vi "BallRollTime.vi"(6 "v_ini":dbl, 8 "error in (no error)":errorcluster, 9 "distance":dbl, 10 "Ball":refnum<class "Ball.lvclass">, 11 "Utilities in":refnum<class "Utilities.lvclass">) -> (0 "error out":errorcluster, 2 "time":dbl, 3 "Utilities out":refnum<class "Utilities.lvclass">)   [LabVIEW 2023, in "Utilities.lvclass"]
uses:
  Utilities.lvclass
  Ball_class/Ball.lvclass
  Ball_class/Ball.lvclass/Ball.ctl
  Ball_class/Read acc_roll.vi
  Ball_class/Read acc_slide.vi
  Ball_class/Read k_switch.vi
  Ball_class/Read velocityNorm.vi
  <vilib>/Analysis/_algsub.llb/Vector Norm.vi
  <vilib>/Analysis/_algsub.llb/Real Vector Norm.vi
panel:
  in  "k_switch":dbl=0.7142857142857143
  in  "acc_slide":dbl=-2.5
  in  "acc_roll":dbl=-0.3
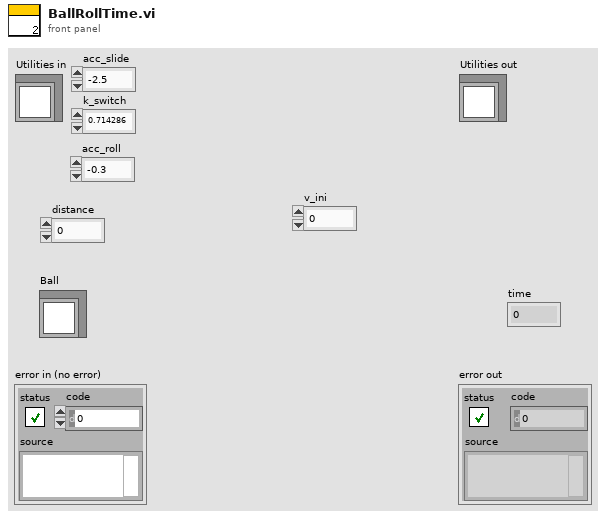
[diagram p1: front panel]
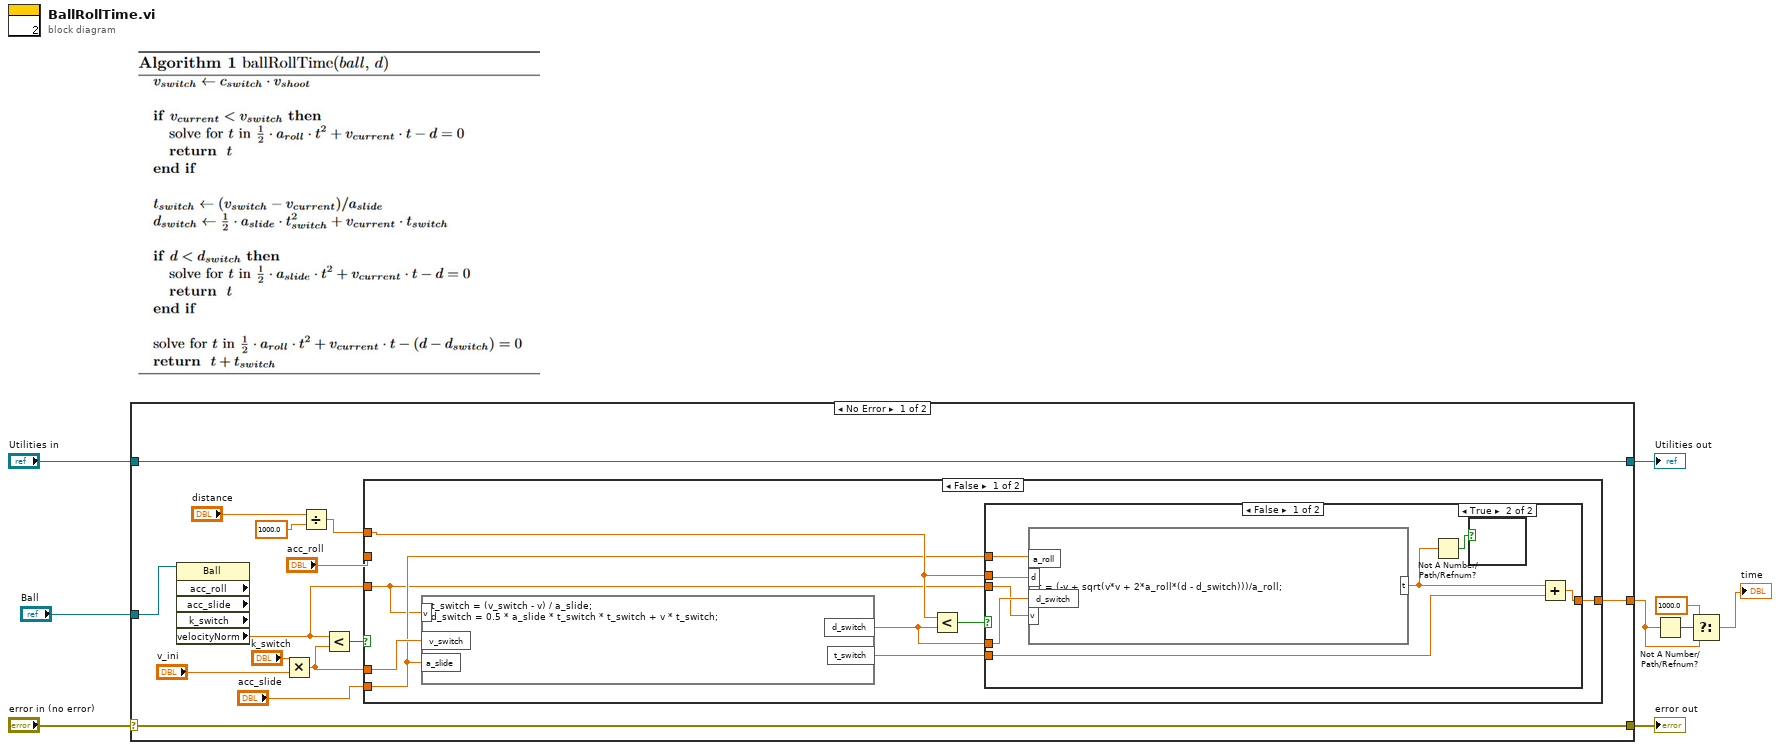
[diagram p0: block diagram]
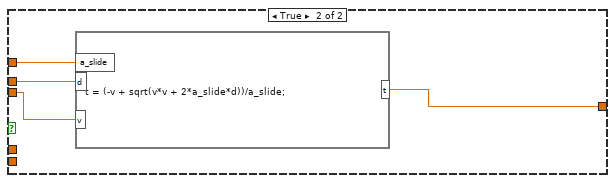
[diagram p3: hidden frame]
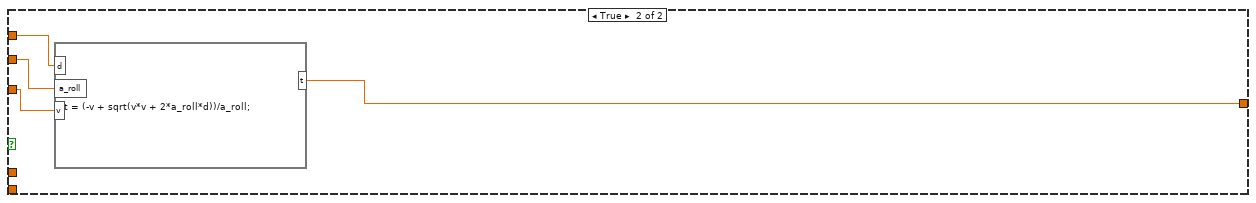
[diagram p4: hidden frame]
diagram:
  n1 = case shown="No Error" "error in (no error)" {
    selector: "error in (no error)" -> [w22 w49]
    tunnel: [w22 w49] -> w8
    tunnel: [w23 w48] -> w6
    tunnel: "Utilities in" -> [w23 w48]
    tunnel: "Ball" -> [w21 _]
    tunnel: [w19 _] -> w2
    frame No Error {
      n2 = property class="Ball" props=["acc_roll", "acc_slide", "k_switch", "velocityNorm"](reference=w21) -> ("velocityNorm"=w18:dbl)  [unwired: 1 in, 5 out]
      n3 = Multiply(x="k_switch", y="v_ini") -> (x*y=w17:dbl)
      n4 = Divide(x="distance", y=1000.0) -> (x/y=w16:dbl)
      n5 = Less?(x=w18, y=w17) -> (x < y?=w20:bool)
      n6 = case shown="False" w20 {
        tunnel: w18 -> [w24 w47]
        tunnel: "acc_roll" -> [_ w46]
        tunnel: w16 -> [w29 w45]
        tunnel: [w28 w44] -> w19
        tunnel: w17 -> [w31 _]
        tunnel: "acc_slide" -> [w27 _]
        frame False {
          n7 = formula code="t_switch = (v_switch - v) / a_slide;\nd_switch = 0.5 * a_slide * t_switch * t_switch + v * t_switch;"("v_switch"=w31, "a_slide"=w27, "v"=w24) -> ("t_switch"=w25:dbl, "d_switch"=w26:dbl)
          n8 = Less?(x=w29, y=w26) -> (x < y?=w30:bool)
          n9 = case shown="False" w30 {
            tunnel: w29 -> [w38 w43]
            tunnel: w27 -> [w37 w42]
            tunnel: w24 -> [w36 w41]
            tunnel: [w34 w40] -> w28
            tunnel: w26 -> [w39 _]
            tunnel: w25 -> [w35 _]
            frame False {
              n10 = formula code="t = (-v + sqrt(v*v + 2*a_roll*(d - d_switch)))/a_roll;"("v"=w36, "a_roll"=w37, "d"=w38, "d_switch"=w39) -> ("t"=w33:dbl)
              n11 = Not A Number/Path/Refnum?(number/path/refnum=w33) -> (NaN/Path/Refnum?=w32:bool)
              n12 = case shown="True" w32 {
                frame False {
                }
                frame True {
                }
              }
              n13 = Add(x=w33, y=w35) -> (x+y=w34:dbl)
            }
            frame True {
              n14 = formula code="t = (-v + sqrt(v*v + 2*a_slide*d))/a_slide;"("v"=w41, "a_slide"=w42, "d"=w43) -> ("t"=w40:dbl)
            }
          }
        }
        frame True {
          n15 = formula code="t = (-v + sqrt(v*v + 2*a_roll*d))/a_roll;"("v"=w47, "a_roll"=w46, "d"=w45) -> ("t"=w44:dbl)
        }
      }
    }
    frame Error {
    }
  }
  "error out" <- w8
  "Utilities out" <- w6
  n16 = Not A Number/Path/Refnum?(number/path/refnum=w2) -> (NaN/Path/Refnum?=w4:bool)
  n17 = Select(t=1000.0, s=w4, f=w2) -> (s? t:f=→"time":dbl)
